vi "CloseQueue.vi"(8 "ErrorArray":errorcluster[](array[cluster])) -> (0 "ErrorArray 2":errorcluster[](array[cluster]))   [LabVIEW 2018, in "Queue.lvlib"]
uses:
  Queue.lvlib
  <userlib>/NIST/NISTErrorLib/NISTErrorLib.lvlib
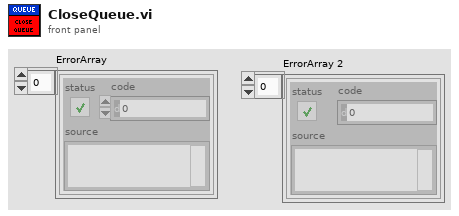
[diagram p1: front panel]
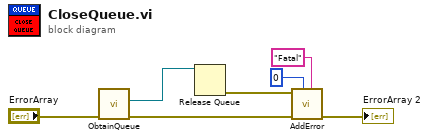
[diagram p0: block diagram]
diagram:
  n1 = call "ObtainQueue.vi"("ErrorArray"="ErrorArray") -> ("ErrorArray"=w1:errorcluster[], "QueueRef"=w3:refnum<queue>)  [unwired: 9 in]
  n2 = Release Queue(queue=w3) -> (error out=w4:errorcluster)  [unwired: 2 in, 2 out]
  n3 = call <userlib>:"AddError.vi"("Severity"="Fatal", "Priority"=u8 0, "ErrorArray"=w1, "error in (no error)"=w4) -> ("ErrorArray"=→"ErrorArray 2":errorcluster[])  [unwired: 6 in, 1 out]
